vi "EditorThumbnail shiftArray.vi"(7 "add":i32, 8 "error in (no error)":errorcluster, 11 "EditorThumbnail in":refnum<class "EditorThumbnail.lvclass">=refnum) -> (0 "error out":errorcluster, 3 "EditorThumbnail out":refnum<class "EditorThumbnail.lvclass">)   [LabVIEW 2018, in "EditorThumbnail.lvclass"]
uses:
  EditorThumbnail.lvclass
  EditorThumbnail.lvclass/EditorThumbnail.ctl
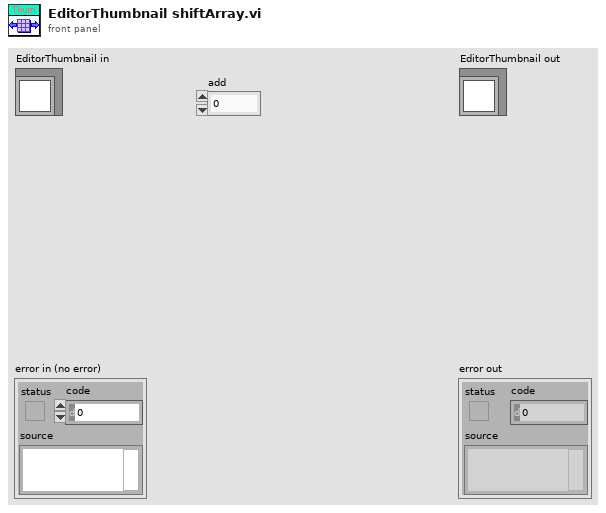
[diagram p1: front panel]
types:
  T1 = cluster{"index":u32, "data":cluster{"xdata":dbl[], "ydata":sgl[]}[], "peak":dbl[], "picture":picture}[]
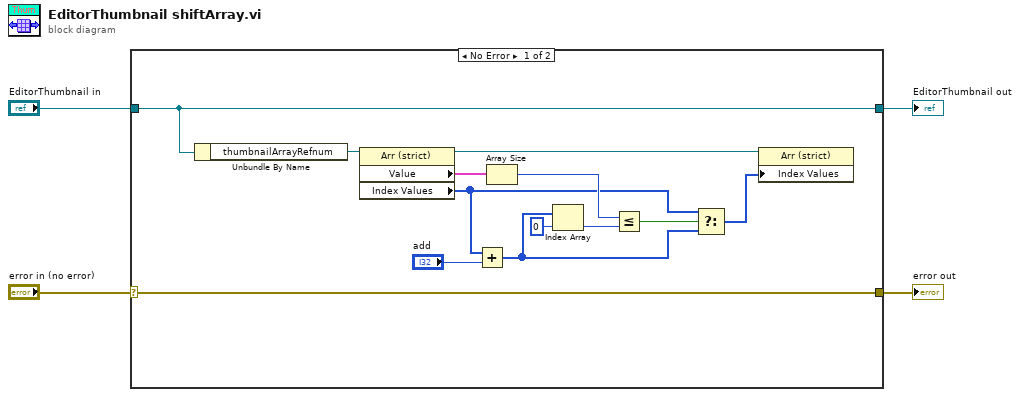
[diagram p0: block diagram]
diagram:
  n1 = case shown="No Error" "error in (no error)" {
    selector: "error in (no error)" -> [w17 w19]
    tunnel: [w17 w19] -> w3
    tunnel: [w16 w18] -> w1
    tunnel: "EditorThumbnail in" -> [w16 w18]
    frame No Error {
      n2 = Unbundle By Name(w16) -> ("thumbnailArrayRefnum"=w15:refnum<vi>)
      n3 = property class="Arr (strict)"(reference=w15) -> (reference out=w13:refnum<vi>, "Value"=w12:T1, "Index Values"=w5:u32[])  [unwired: 1 in, 1 out]
      n4 = Add(x=w5, y="add") -> (x+y=w6:u32[])
      n5 = Array Size(array=w12) -> (size(s)=w11:i32)
      n6 = Index Array(array=w6, index=0) -> (element=w10:u32)
      n7 = Less Or Equal?(x=w11, y=w10) -> (x <= y?=w9:bool)
      n8 = Select(t=w5, s=w9, f=w6) -> (s? t:f=w8:u32[])
      n9 = property class="Arr (strict)"(reference=w13, "Index Values"=w8) -> ()  [unwired: 1 in, 2 out]
    }
    frame Error {
    }
  }
  "error out" <- w3
  "EditorThumbnail out" <- w1
